vi "dashOffset.vi"(8 "Error In":errorcluster, 11 "QPen In":refnum<class "QPen.lvclass">) -> (0 "Error Out":errorcluster, 2 "Value":dbl, 3 "QPen Out":refnum<class "QPen.lvclass">)   [LabVIEW 2014, in "QPen.lvclass"]
doc: "LabVIEW-specific documentation is not yet available. See <b>http://doc.qt.io/qt-5/QPen.html#dashOffset</b>"
uses:
  QPen.lvclass
  LQ Core/LQSerialData/LQSerialData.lvclass/LQSerialData.ctl
  LQ Core/LQ Core.lvlib
  LQ Core/LQSerialData/LQSerialData.lvclass
panel:
  # "Copyright (c) 2016 Sze Howe Koh\n\nThis Source Code Form is subject to the terms of the Mozilla Public\nLicense, v. 2.0. If a copy of the MPL was not distributed with this\nfile, You can obtain one at http://mozilla.org/MPL/2.0/."
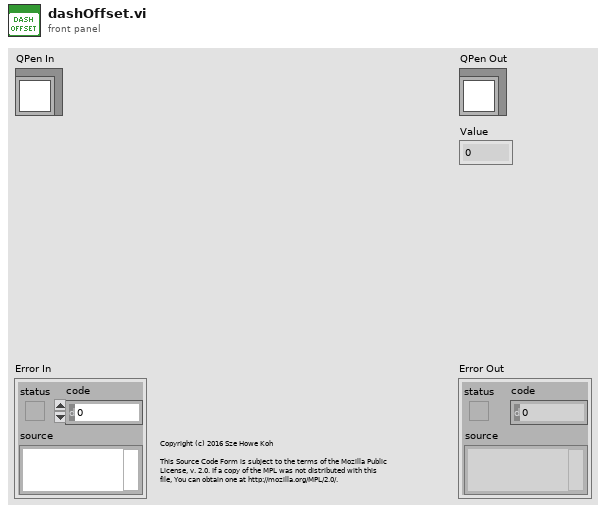
[diagram p1: front panel]
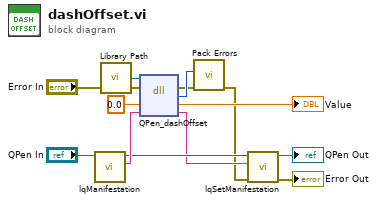
[diagram p0: block diagram]
diagram:
  n1 = call "lqManifestation.vi"("LQSerialData in"="QPen In") -> ("Manifestation"=w10:string, "LQSerialData out"=w8:refnum<class "QPen.lvclass">)  [unwired: 9 in]
  n2 = call "Library Path.vi"() -> ("Library Path"=w5:path)
  n3 = dll-call lib="?" fn="QPen_dashOffset"(path in=w5, error in="Error In", "_retVal"=0.0 ("retVal"), "_instance"=w10) -> (error out=w2:errorcluster, w3:i32, "_retVal"=→"Value":dbl, "_instance"=w6:string)  [unwired: 1 in, 1 out]
  n4 = call "Pack Errors.vi"("Error In"=w2, "Error Code"=w3) -> ("Error Out"=w1:errorcluster)  [unwired: 9 in]
  n5 = call "lqSetManifestation.vi"("Error In"=w1, "Manifestation"=w6, "LQSerialData in"=w8) -> ("Error Out"=→"Error Out":errorcluster, "LQSerialData out"=→"QPen Out":refnum<class "QPen.lvclass">)  [unwired: 7 in]
